vi "View.vi"(8 "error in (no error)":errorcluster, 11 "XY Stage Class in":refnum<class "XY Stage Class.lvclass">) -> (0 "error out":errorcluster, 3 "XY Stage Class out":refnum<class "XY Stage Class.lvclass">)   [LabVIEW 2022 SP3, in "XY Stage Class.lvclass"]
uses:
  XY Stage Class.lvclass
  C:/XY Stage/iView/base view/base view.lvclass
  Interfaces/2-Axis Stage API/2-Axis Stage Async API.lvclass
  XY Controller/XY Stage Controller/XY Stage Controller.lvclass
  C:/XY Stage/XY Stage/Interfaces/2-Axis Stage API/2-Axis Stage Async API.lvclass
  iView/base view/Accessors/Read Event Registration Refnum.vi
  iView/base view/Accessors/Read View Refnum.vi
  iView/base view/base view.lvclass
panel:
  in  "2-Axis Stage":refnum<class "2-Axis Stage Async API.lvclass">
  out "XY Position Graph":cluster{"X":dbl, "Y":dbl}[](graph)
  in  "Abort Motion":bool
  in  "Home Stage":bool
  in  "Move Stage":bool
  in  "Y-Destination":dbl min=-100.0 max=100.0
  in  "X-Destination":dbl min=-100.0 max=100.0
  in  "Clear Error":bool
  in  "Set X-Speed":u16
  in  "Set Y-Speed":u16
  in  "Set X-Acceleration":u16
  in  "Set Y-Acceleration":u16
  out "X-Speed":dbl
  out "Y-Speed":dbl
  out "X-Current Speed":dbl
  out "Y-Current Speed":dbl
  out "X-Acceleration":dbl
  out "Y-Acceleration":dbl
  out "Y-Homed":bool
  out "X-Homed":bool
  out "X-Moving":bool
  out "Y-Moving":bool
  out "Y-Position":dbl
  out "X-Position":dbl
  out "Stage Error":errorcluster
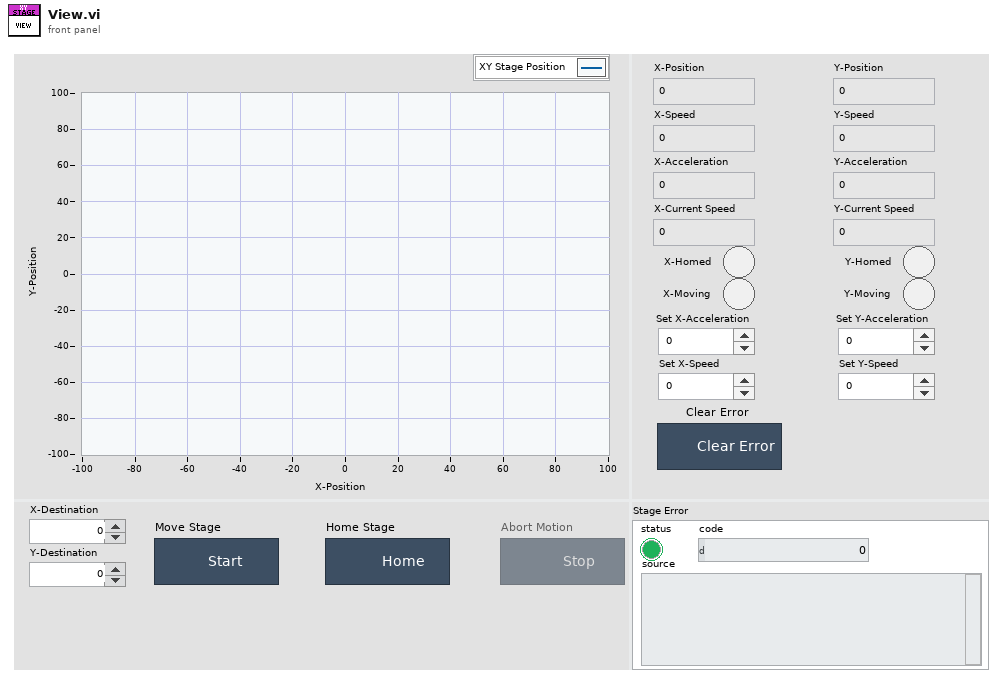
[diagram p1: front panel]
types:
  T1 = typedef "base view.lvclass/Events.ctl" = cluster{"Open":refnum<user-event>, "Close":refnum<user-event>, "Hide":refnum<user-event>}
  T2 = enum32{"Invalid", "Standard", "Closed", "Hidden", "Minimized", "Maximized"}
  T3 = enum32{"invalid app kind", "Development System", "Run Time System", "Student Edition", "Embedded LabVIEW", "Evaluation", "Custom"}
  T4 = enum8{"Enabled", "Disabled", "Disabled and Grayed Out"}
  T5 = cluster{"Current Position X":dbl, "Current Position Y":dbl}[]
  T6 = cluster{"Core":cluster{"Current VI Reference":refnum<vi>, "Close Panel on Exit?":bool}, "2-Axis Stage":refnum<class "2-Axis Stage Async API.lvclass">}
  T7 = cluster{"Current VI Reference":refnum<vi>, "Close Panel on Exit?":bool}
  T8 = cluster{"Event Registration Refnum":refnum<event-registration>, "Event Registration Refnum":refnum<event-registration>}
  T9 = cluster{"Event Registration Refnum":refnum<event-registration>, "Event Registration Refnum":refnum<event-registration>, "Event Registration Refnum":refnum<event-registration>}
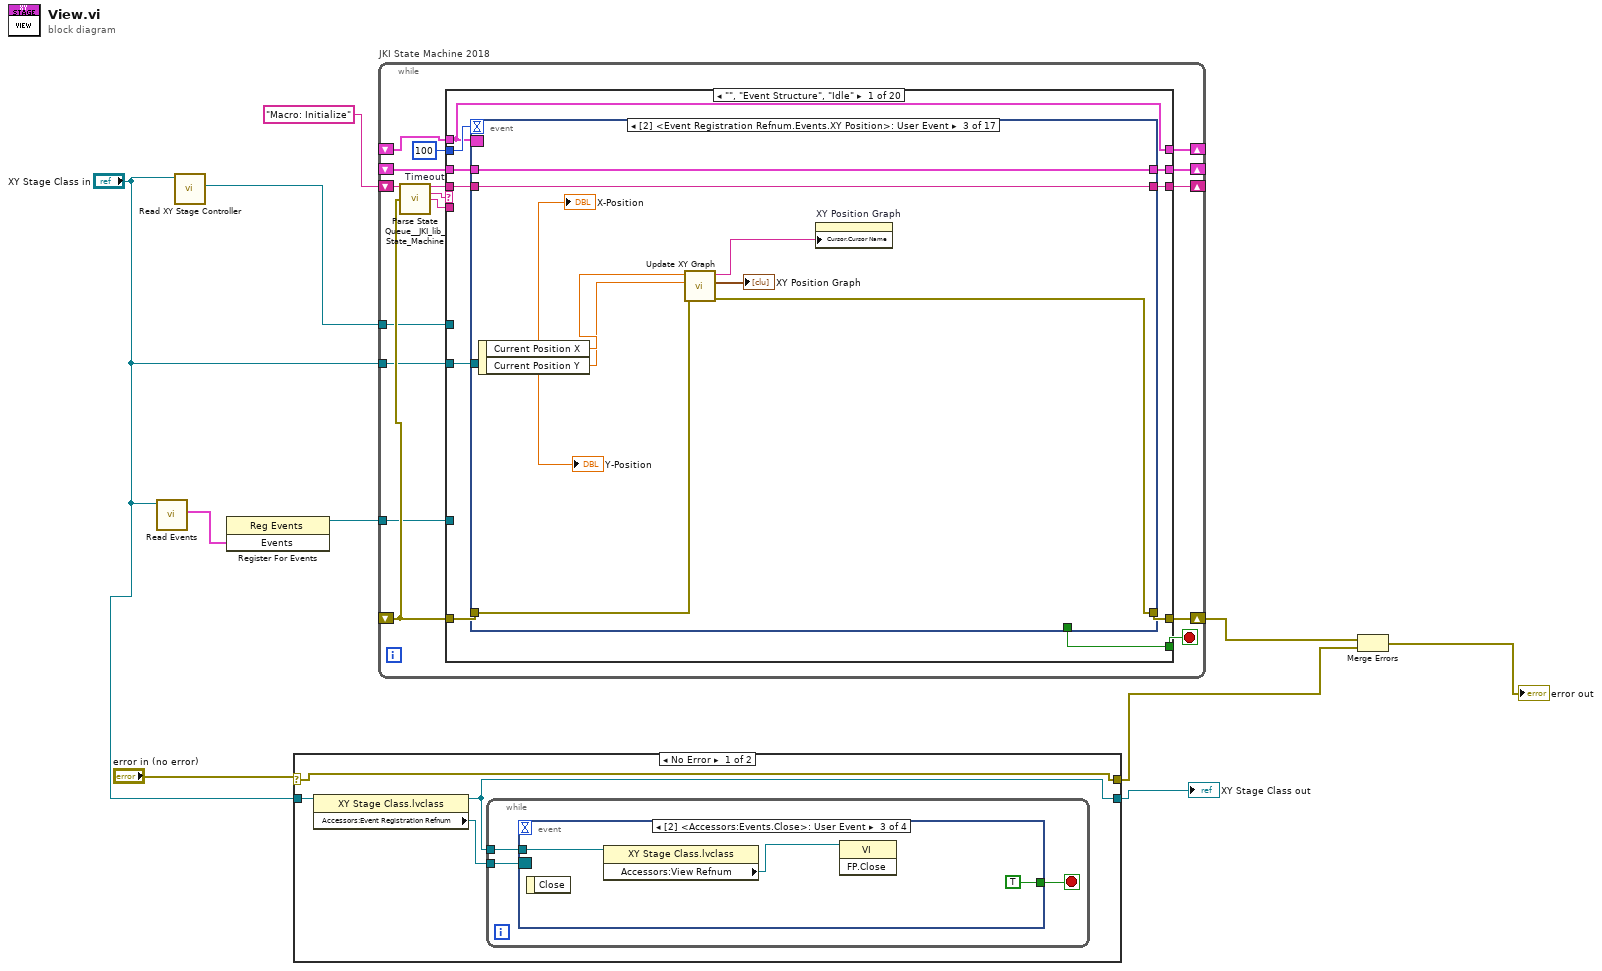
[diagram p0: block diagram]
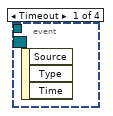
[diagram p2: hidden frame]
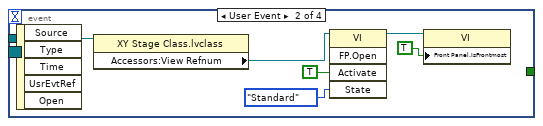
[diagram p3: hidden frame]
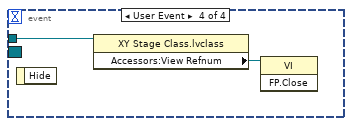
[diagram p4: hidden frame]
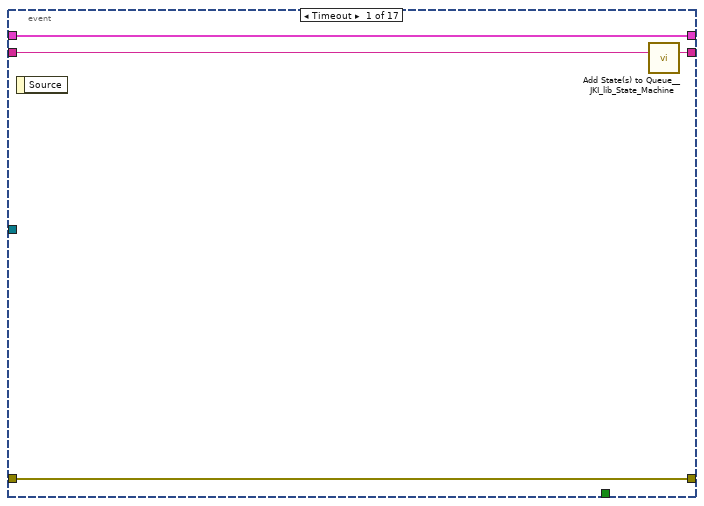
[diagram p6: hidden frame]
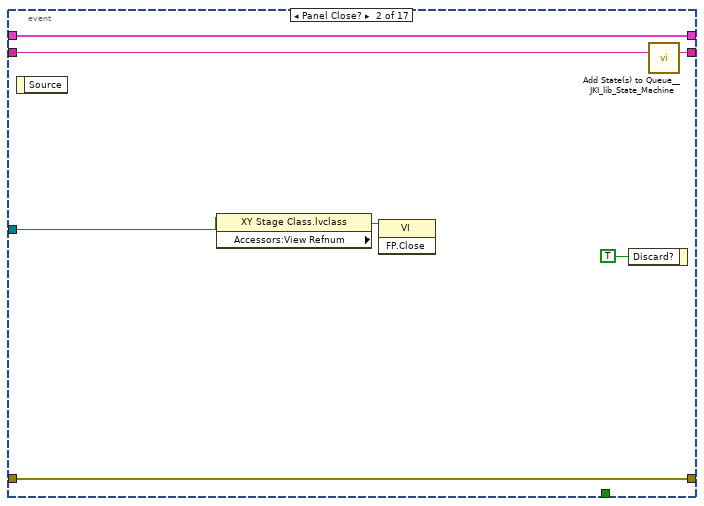
[diagram p7: hidden frame]
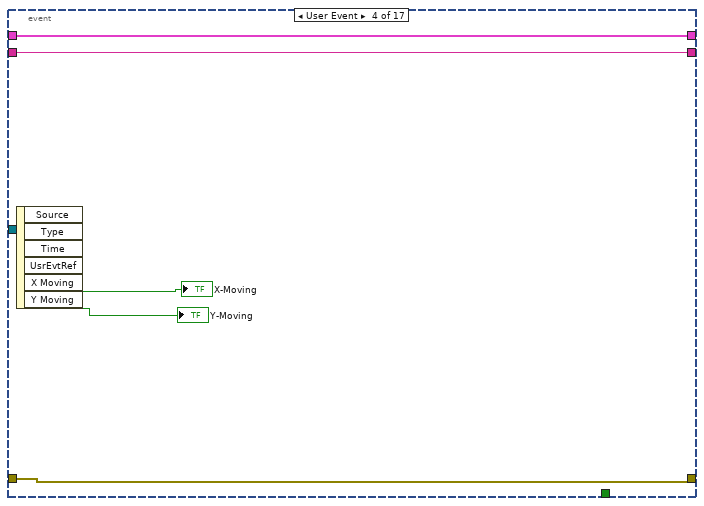
[diagram p8: hidden frame]
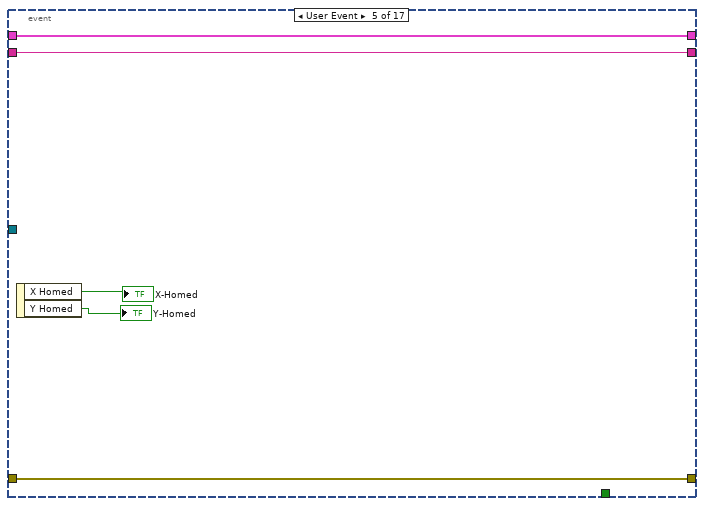
[diagram p9: hidden frame]
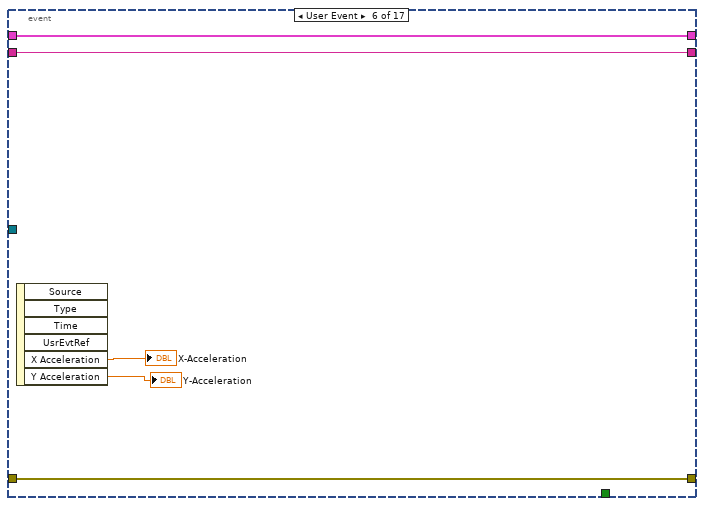
[diagram p10: hidden frame]
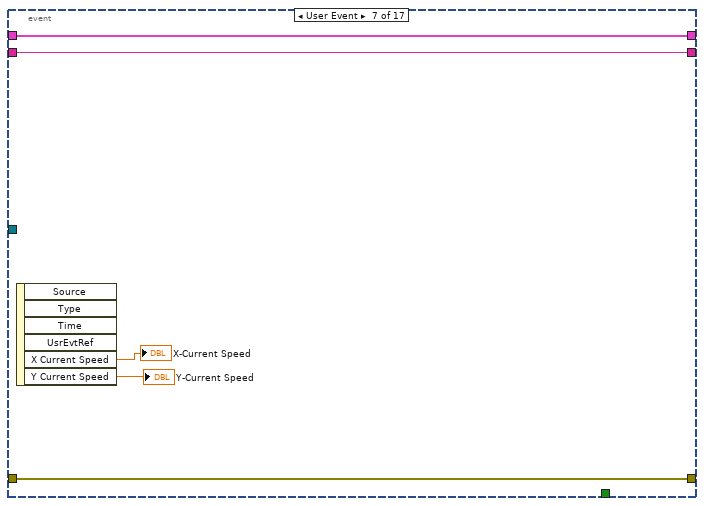
[diagram p11: hidden frame]
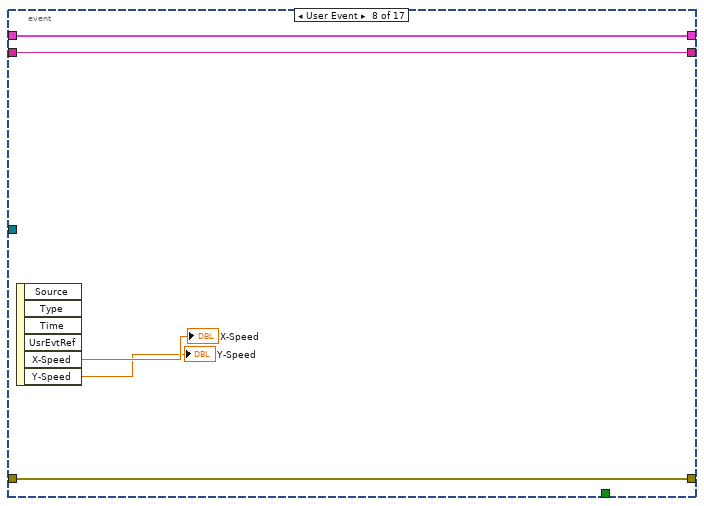
[diagram p12: hidden frame]
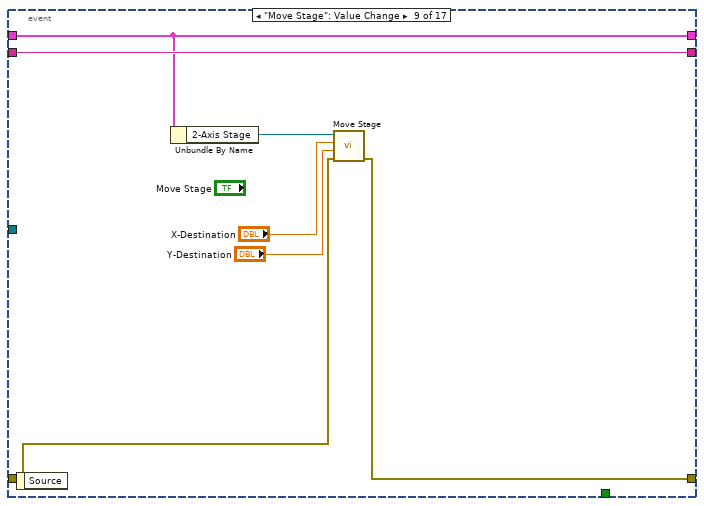
[diagram p13: hidden frame]
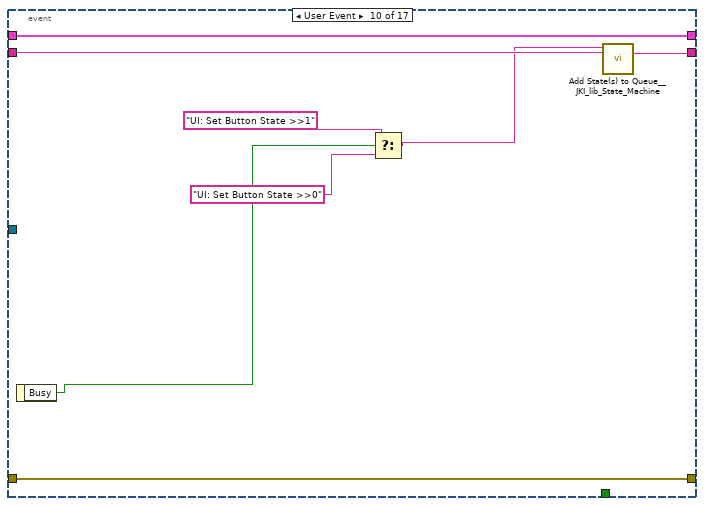
[diagram p14: hidden frame]
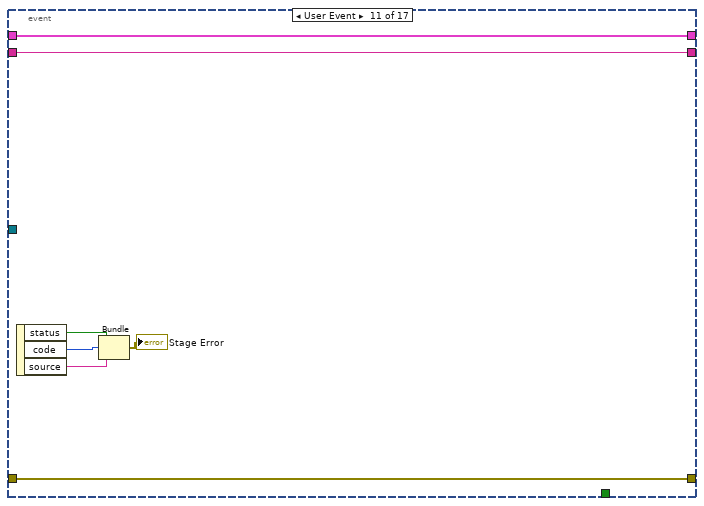
[diagram p15: hidden frame]
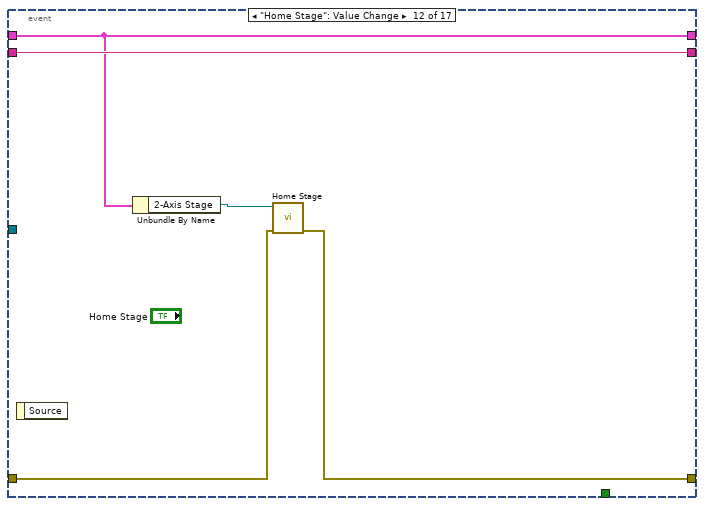
[diagram p16: hidden frame]
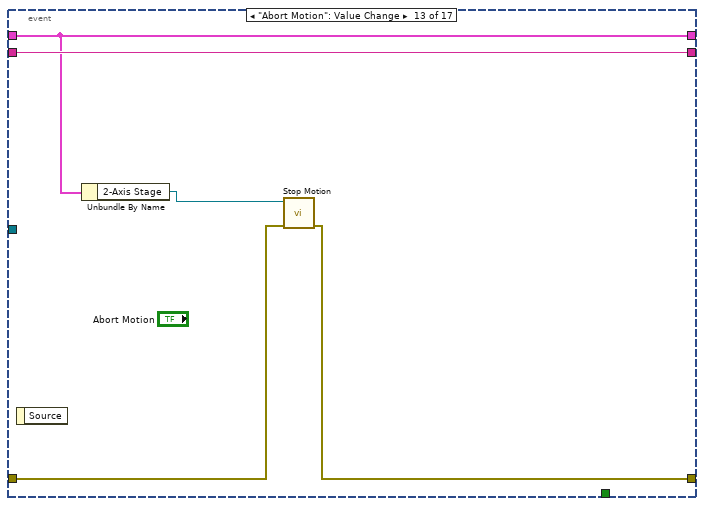
[diagram p17: hidden frame]
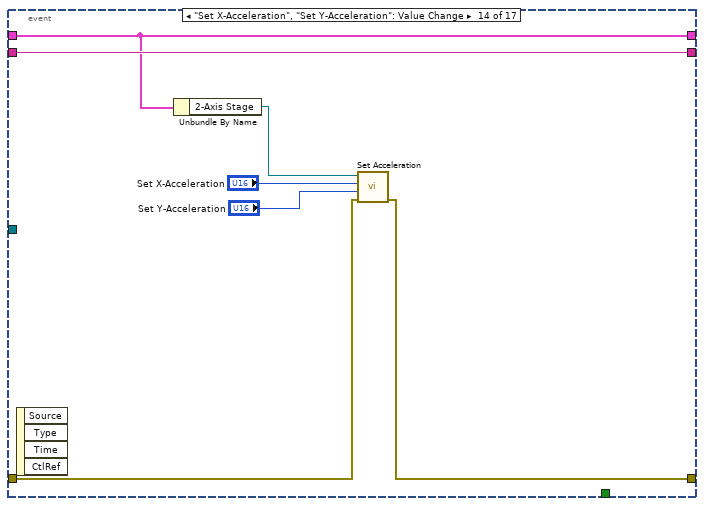
[diagram p18: hidden frame]
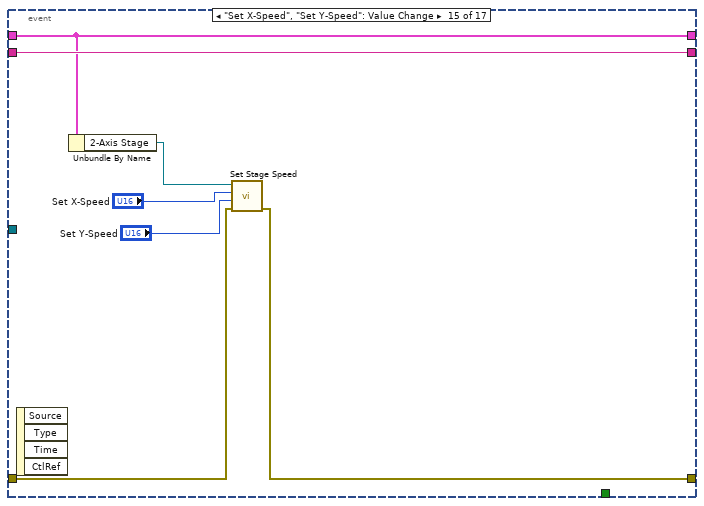
[diagram p19: hidden frame]
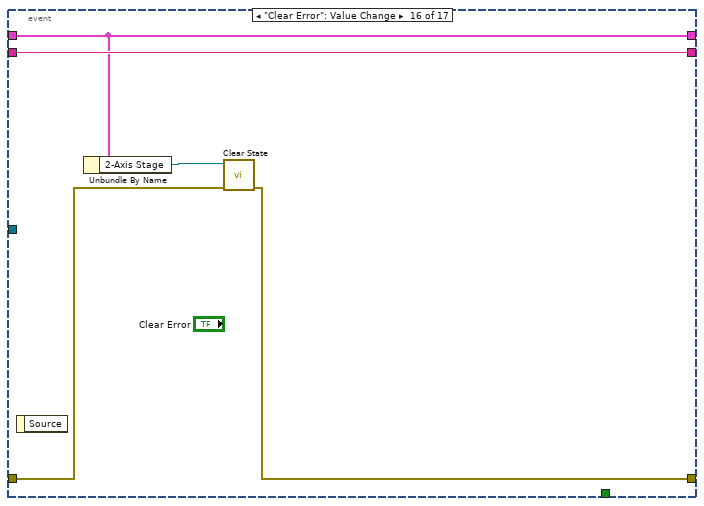
[diagram p20: hidden frame]
diagram:
  n1 = call "Read Events.vi"("In"="XY Stage Class in") -> ("Events"=w7:T1)  [unwired: 8 in, 2 out]
  n2 = call "Read XY Stage Controller.vi"("In"="XY Stage Class in") -> ("XY Stage Controller"=w8:refnum<class "XY Stage Controller.lvclass">)  [unwired: 8 in, 2 out]
  n3 = register-events(w7) -> (reference out=w6:refnum<event-registration>)  [unwired: 2 in, 1 out]
  n4 = case shown="No Error" "error in (no error)" {
    selector: "error in (no error)" -> [w14 w30]
    tunnel: [w14 w30] -> w3
    tunnel: [w11 w29] -> w10
    tunnel: "XY Stage Class in" -> [w13 w29]
    frame No Error {
      n5 = property class="XY Stage Class.lvclass"(reference=w13) -> (reference out=w11:refnum<class "XY Stage Class.lvclass">, "Accessors:Event Registration Refnum"=w12:refnum<event-registration>)  [unwired: 1 in, 1 out]
      n6 = while {
        tunnel: w12 -> [w17]
        tunnel: w11 -> [w15]
        stop <- w16 stop-if-true
        n7 = event shown="[2] <Accessors:Events.Close>: User Event" {
          selector: w17 -> [_ _ _ _]
          dyn-events: _ -> [_ _ _ _]
          timeout: _ -> [_ _ _ _]
          tunnel: [_ _ TRUE _] -> w16
          tunnel: w15 -> [_ w23 w24 w28]
          event Timeout {
            n8 = event-data() -> ()  [unwired: 1 in, 3 out]
          }
          event User Event {
            n9 = event-data() -> ()  [unwired: 1 in, 5 out]
            n10 = property class="XY Stage Class.lvclass"(reference=w23) -> ("Accessors:View Refnum"=w22:refnum<vi>)  [unwired: 1 in, 2 out]
            n11 = invoke class="VI" method="FP.Open"(reference=w22, "Activate"=TRUE ("Activate?"), "State"=T2."Standard") -> (reference out=w19:refnum<vi>)  [unwired: 2 in, 4 out]
            n12 = property class="VI"(reference=w19, "Front Panel.IsFrontmost"=TRUE ("Front Panel Window:Is Frontmost")) -> ()  [unwired: 1 in, 2 out]
          }
          event User Event {
            n13 = event-data() -> ()  [unwired: 1 in, 1 out]
            n14 = property class="XY Stage Class.lvclass"(reference=w24) -> ("Accessors:View Refnum"=w25:refnum<vi>)  [unwired: 1 in, 2 out]
            n15 = invoke class="VI" method="FP.Close"(reference=w25) -> ()  [unwired: 2 in, 3 out]
          }
          event User Event {
            n16 = event-data() -> ()  [unwired: 1 in, 1 out]
            n17 = property class="XY Stage Class.lvclass"(reference=w28) -> ("Accessors:View Refnum"=w27:refnum<vi>)  [unwired: 1 in, 2 out]
            n18 = invoke class="VI" method="FP.Close"(reference=w27) -> ()  [unwired: 2 in, 3 out]
          }
        }
      }
    }
    frame Error {
    }
  }
  "XY Stage Class out" <- w10
  n19 = while "JKI State Machine 2018" {
    shift-right: [w39] -> _
    shift-left: _ -> [w38]
    shift-right: [w42] -> w4
    shift-left: _ -> [w36]
    shift-right: [w41] -> _
    shift-left: "Macro: Initialize" -> [w43]
    shift-right: [w35] -> _
    shift-left: _ -> [w34]
    tunnel: w8 -> [w33]
    tunnel: w6 -> [w32]
    tunnel: "XY Stage Class in" -> [w31]
    stop <- w40 stop-if-true
    w37 = 100  # Timeout
    n20 = call <vilib>:"Parse State Queue__JKI_lib_State_Machine.vi"("State Queue"=w43, "Error In (no error)"=w36) -> ("Remaining States"=w45:string, "Current State"=w46:string, "Arguments"=w44:string)  [unwired: 11 in]
    n21 = case shown="\"\", \"Event Structure\", \"Idle\"" w46 {
      selector: w46 -> [_ _ w162 _ _ _ _ _ _ _ _ _ _ _ _ _ _ _ _ _]
      tunnel: w45 -> [w56 w160 w166 w186 w193 w199 w204 w213 w220 w225 w248 w259 w291 w313 w325 w395 w401 w412 w417 w427]
      tunnel: w44 -> [_ _ _ _ _ _ _ _ _ _ _ _ w280 w308 w319 _ _ _ _ _]
      tunnel: w38 -> [w54 w157 w164 w179 w190 w197 w201 _ w215 w222 w245 w263 w282 w311 w321 w392 w398 w409 w414 w426]
      tunnel: [w53 w158 w168 w183 errorcluster {"status"=FALSE, "code"=0, "source"=""} ("error out") w196 w202 w210 w216 w223 w230 w254 w277 w309 w322 w393 w399 w410 w415 w423] -> w42
      tunnel: w36 -> [w52 w158 w167 w183 w187 w196 w202 w210 w217 w223 w237 w261 w276 w310 w323 w393 w399 w410 w415 w424]
      tunnel: [w55 w159 w165 w185 w192 w198 w203 w212 w219 w224 w247 w260 w291 w312 w324 w394 w400 w411 w416 w427] -> w41
      tunnel: [w48 _ _ _ _ TRUE _ _ _ _ _ _ _ _ _ _ _ _ _ _] -> w40
      tunnel: [w51 w157 w164 w184 w190 w197 w201 w206 w215 w222 w245 w263 w282 w311 w321 w392 w398 w409 w414 w426] -> w39
      tunnel: w37 -> [w50 _ _ _ _ _ _ _ _ _ _ _ _ _ _ _ _ _ _ _]
      tunnel: [w49 w156 w161 w173 w188 w194 w200 w207 w214 w221 w246 w274 w283 w307 w318 w391 w397 w402 w413 w421] -> w35
      tunnel: w34 -> [w49 w156 w161 w173 w188 w194 w200 w207 w214 w221 w246 w274 w283 w307 w318 w391 w397 w402 w413 _]
      tunnel: w33 -> [_ _ _ _ _ _ _ w205 _ _ _ _ _ _ _ _ _ _ _ _]
      tunnel: w32 -> [_ _ _ _ _ _ _ _ _ _ _ _ _ _ _ _ _ _ _ w422]
      tunnel: w31 -> [w47 _ _ _ _ _ _ _ _ _ _ _ _ _ _ _ _ _ _ _]
      frame "", "Event Structure", "Idle" {
        n22 = event shown="[2] <Event Registration Refnum.Events.XY Position>: User Event" {
          selector: w49 -> [_ _ _ _ _ _ _ _ _ _ _ _ _ _ _ _ _]
          dyn-events: _ -> [_ _ _ _ _ _ _ _ _ _ _ _ _ _ _ _ _]
          timeout: w50 -> [_ _ _ _ _ _ _ _ _ _ _ _ _ _ _ _ _]
          tunnel: w56 -> [w60 w67 w74 w80 w85 w90 w95 w100 w107 w112 w122 w127 w132 w139 w146 w151 w155]
          tunnel: [w59 w66 w74 w80 w85 w90 w95 w100 w107 w113 w122 w127 w132 w139 w146 w151 w155] -> w55
          tunnel: w54 -> [w57 w64 w75 w79 w84 w89 w94 w99 w106 w115 w121 w126 w131 w138 w145 w150 w154]
          tunnel: [w58 w65 w68 w76 w81 w86 w91 w96 w101 w114 w116 w123 w129 w133 w142 w147 w152] -> w53
          tunnel: w52 -> [w58 w65 w69 w76 w81 w86 w91 w96 w102 w114 w116 w124 w128 w134 w143 w148 w152]
          tunnel: [w57 w64 w75 w79 w84 w89 w94 w99 w106 w115 w121 w126 w131 w138 w145 w150 w154] -> w51
          tunnel: [_ _ _ _ _ _ _ _ _ _ _ _ _ _ _ _ TRUE] -> w48
          tunnel: w47 -> [_ w61 _ _ _ _ _ _ _ _ _ _ _ _ _ _ _]
          event Timeout {
            n23 = event-data() -> ()  [unwired: 1 in, 1 out]
            n24 = call <vilib>:"Add State(s) to Queue__JKI_lib_State_Machine.vi"("State(s) in (\"\")"=w60) -> ("States Out"=w59:string)  [unwired: 14 in]
          }
          event Panel Close? {
            n25 = event-data() -> ()  [unwired: 1 in, 1 out]
            n26 = property class="XY Stage Class.lvclass"(reference=w61) -> ("Accessors:View Refnum"=w62:refnum<vi>)  [unwired: 1 in, 2 out]
            n27 = invoke class="VI" method="FP.Close"(reference=w62) -> ()  [unwired: 2 in, 3 out]
            n28 = event-data("Discard?"=TRUE) -> ()  [unwired: 1 in, 1 out]
            n29 = call <vilib>:"Add State(s) to Queue__JKI_lib_State_Machine.vi"("State(s) in (\"\")"=w67) -> ("States Out"=w66:string)  [unwired: 14 in]
          }
          event User Event {
            n30 = event-data() -> ("Current Position X"=w72:dbl, "Current Position Y"=w71:dbl)  [unwired: 1 in]
            "Y-Position" <- w71
            "X-Position" <- w72
            n31 = call "Update XY Graph.vi"("error in (no error)"=w69, "Current Position Y"=w71, "Current Position X"=w72) -> ("error out"=w68:errorcluster, "Array"=→"XY Position Graph":T5, "String"=w70:string)  [unwired: 6 in]
            n32 = property on="XY Position Graph" class="XYGraph (strict)"("Cursor.Cursor Name"=w70) -> ()  [unwired: 2 in, 2 out]
          }
          event User Event {
            n33 = event-data() -> ("X Moving"=→"X-Moving":bool, "Y Moving"=→"Y-Moving":bool)  [unwired: 1 in, 4 out]
          }
          event User Event {
            n34 = event-data() -> ("X Homed"=→"X-Homed":bool, "Y Homed"=→"Y-Homed":bool)  [unwired: 1 in]
          }
          event User Event {
            n35 = event-data() -> ("X Acceleration"=→"X-Acceleration":dbl, "Y Acceleration"=→"Y-Acceleration":dbl)  [unwired: 1 in, 4 out]
          }
          event User Event {
            n36 = event-data() -> ("X Current Speed"=→"X-Current Speed":dbl, "Y Current Speed"=→"Y-Current Speed":dbl)  [unwired: 1 in, 4 out]
          }
          event User Event {
            n37 = event-data() -> ("X-Speed"=→"X-Speed":dbl, "Y-Speed"=→"Y-Speed":dbl)  [unwired: 1 in, 4 out]
          }
          event "Move Stage": Value Change {
            n38 = event-data() -> ()  [unwired: 1 in, 1 out]
            n39 = Unbundle By Name(w106) -> ("2-Axis Stage"=w105:refnum<class "2-Axis Stage Async API.lvclass">)
            n40 = call-dynamic "Move Stage.vi"("error in (no error)"=w102, "Y Axis"="Y-Destination", "X Axis"="X-Destination", "2-Axis Stage in"=w105) -> ("error out"=w101:errorcluster)  [unwired: 6 in, 1 out]
          }
          event User Event {
            n41 = event-data() -> ("Busy"=w111:bool)  [unwired: 1 in]
            n42 = Select(t="UI: Set Button State >>1", s=w111, f="UI: Set Button State >>0") -> (s? t:f=w108:string)
            n43 = call <vilib>:"Add State(s) to Queue__JKI_lib_State_Machine.vi"("State(s) in Front (\"\")"=w108, "State(s) in (\"\")"=w112) -> ("States Out"=w113:string)  [unwired: 13 in]
          }
          event User Event {
            n44 = event-data() -> ("status"=w120:bool, "code"=w119:i32, "source"=w118:string)  [unwired: 1 in]
            n45 = Bundle("status"=w120, "code"=w119, "source"=w118) -> (→"Stage Error":errorcluster)  [unwired: 1 in]
          }
          event "Home Stage": Value Change {
            n46 = event-data() -> ()  [unwired: 1 in, 1 out]
            n47 = Unbundle By Name(w126) -> ("2-Axis Stage"=w125:refnum<class "2-Axis Stage Async API.lvclass">)
            n48 = call-dynamic "Home Stage.vi"("error in (no error)"=w124, "2-Axis Async Home in"=w125) -> ("error out"=w123:errorcluster)  [unwired: 8 in, 1 out]
          }
          event "Abort Motion": Value Change {
            n49 = event-data() -> ()  [unwired: 1 in, 1 out]
            n50 = Unbundle By Name(w131) -> ("2-Axis Stage"=w130:refnum<class "2-Axis Stage Async API.lvclass">)
            n51 = call-dynamic "Stop Motion.vi"("error in (no error)"=w128, "2-Axis Stage in"=w130) -> ("error out"=w129:errorcluster)  [unwired: 8 in, 1 out]
          }
          event "Set X-Acceleration", "Set Y-Acceleration": Value Change {
            n52 = event-data() -> ()  [unwired: 1 in, 4 out]
            n53 = Unbundle By Name(w138) -> ("2-Axis Stage"=w137:refnum<class "2-Axis Stage Async API.lvclass">)
            n54 = call-dynamic "Set Acceleration.vi"("error in (no error)"=w134, "Y Axis"="Set Y-Acceleration", "X Axis"="Set X-Acceleration", "2-Axis Stage in"=w137) -> ("error out"=w133:errorcluster)  [unwired: 6 in, 1 out]
          }
          event "Set X-Speed", "Set Y-Speed": Value Change {
            n55 = event-data() -> ()  [unwired: 1 in, 4 out]
            n56 = Unbundle By Name(w145) -> ("2-Axis Stage"=w144:refnum<class "2-Axis Stage Async API.lvclass">)
            n57 = call-dynamic "Set Stage Speed.vi"("error in (no error)"=w143, "Y Axis"="Set Y-Speed", "X Axis"="Set X-Speed", "2-Axis Stage in"=w144) -> ("error out"=w142:errorcluster)  [unwired: 6 in, 1 out]
          }
          event "Clear Error": Value Change {
            n58 = event-data() -> ()  [unwired: 1 in, 1 out]
            n59 = Unbundle By Name(w150) -> ("2-Axis Stage"=w149:refnum<class "2-Axis Stage Async API.lvclass">)
            n60 = call-dynamic "Clear State.vi"("error in (no error)"=w148, "2-Axis Stage Status in"=w149) -> ("error out"=w147:errorcluster)  [unwired: 8 in, 1 out]
          }
          event User Event {
            n61 = event-data() -> ()  [unwired: 1 in, 1 out]
          }
        }
      }
      frame "---------- Core ----------" {
        # "Do not put any code in this frame.\n(it is a separator no-op)"
        n62 = call <vilib>:"Add State(s) to Queue__JKI_lib_State_Machine.vi"("State(s) in (\"\")"=w160) -> ("States Out"=w159:string)  [unwired: 14 in]
      }
      frame Default {
        w171 = 42 items=["No error", "Argument error", "Memory is full", "Out of zone", "End of file", "File already open", "Generic file I/O error", "File not found", "File permission error", "Disk is full", "Duplicate path", "Too many files open", "System feature not enabled", "Resource file not found", "Cannot add resource", "Resource not found", "Image not found", "Image memory error", "Pen does not exist", "Config type invalid", "Config token not found", "Config parse error", "Config memory error", "Bad external code format", "Bad external code offset", "External code not present", "Null window", "Destroy window error", "Null menu", "Print aborted", "Bad print record", "Print driver error", "Windows error during printing", "Memory error during printing", "Print dialog error", "Generic print error", "Invalid device refnum", "Device not found", "Device parameter error", "Device unit error", "Cannot open device", "Device call aborted", "Generic error", "Cancelled by user", "Object ID too low", "Object ID too high", "Object not in heap", "Unknown heap", "Unknown object (invalid DefProc)", "Unknown object (DefProc not in table)", "Message out of range", "Invalid (null) method", "Unknown message", "Manager call not supported", "Bad address", "Network operation in progress", "Network operation timed out", "Connection is busy", "Network attribute not supported", "Network error", "Address in use", "System out of memory", "Connection aborted", "Connection refused", "Not connected", "Already connected", "Connection closed", "Initialization error (interapplication manager)", "Bad occurrence", "Wait on unbound occurrence handler", "Occurrence queue overflow", "Datalog type conflict", "Unused", "Unrecognized type (interapplication manager)", "Memory corrupt", "Failed to make temporary DLL", "Old CIN version", "Drag socket not found", "Failed to load drop-object", "Failed to register OLE object", "Failed to release OLE object", "Format specifier type mismatch", "Unknown format specifier", "Too few format specifiers", "Too many format specifiers", "Scan failed", "Newer CIN version", "Error converting to variant", "Runtime menu error", "Password tampered", "Variant attribute not found", "Incompatible variant data type", "Event data is not available", "Event Store is not present", "Occurrence is not found", "Event Queue is not created", "Event info is not available", "Refnum passed is NULL", "Error retrieving Class GUID", "Error retrieving CoClass GUID", "Error retrieving TypeLib GUID.", "Bad built application magic bytes.", "Specific driver is different from the specific driver associated with the Logical Name.", "There is no session opened to the class driver.", "Max Error", "MAX - Error with config objects", "MAX - Error loading configuration", "MAX - Group not supported"]
        # "Current State"
        # "Do not delete, rename, or modify this frame.\n(this is used to capture unhandled states and typos)"
        # "Handle mistyped state name (developer tool)"
        n63 = Format Into String(format string="Software Exception: Unhandled State \"%s\"." ("message"), error in=w167, w162) -> (resulting string=w170:string, error out=w169:errorcluster)  [unwired: 1 in]
        n64 = call <vilib>:"Error Cluster From Error Code.vi"("show call chain? (False)"=TRUE, "error in (no error)"=w169, "error message (\"\")"=w170, "error code (0)"=w171) -> ("error out"=w168:errorcluster)  [unwired: 5 in]
        n65 = call <vilib>:"Add State(s) to Queue__JKI_lib_State_Machine.vi"("State(s) in (\"\")"=w166) -> ("States Out"=w165:string)  [unwired: 14 in]
      }
      frame "Initialize Core Data" {
        # "Do not delete, rename, or modify this frame.\n(this is used to determine panel behavior on exit)"
        # "originally closed?"
        # "exe?"
        # "If panel starts closed or is an EXE, then close it when we exit"
        n66 = property class="VI"() -> ("FP.State"=w176:T2)  [unwired: 2 in, 2 out]
        n67 = property class="App"() -> ("App.Kind"=w182:T3)  [unwired: 2 in, 2 out]
        n68 = control-ref of="Current VI Reference"() -> (w177:refnum<vi>)
        n69 = Equal?(x=w176, y=T2."Closed" ("Front Panel Window:State")) -> (x = y?=w174:bool)
        n70 = Equal?(x=w182, y=T3."Run Time System" ("Application:Kind")) -> (x = y?=w180:bool)
        n71 = Or(x=w174, y=w180) -> (x .or. y?=w178:bool)
        n72 = Bundle By Name(cluster=w179, "Core.Current VI Reference"=w177, "Core.Close Panel on Exit?"=w178) -> (w184:T6)
        n73 = call <vilib>:"Add State(s) to Queue__JKI_lib_State_Machine.vi"("State(s) in (\"\")"=w186) -> ("States Out"=w185:string)  [unwired: 14 in]
      }
      frame "Error Handler" {
        # "Handle any errors here.\nYou can also output any states to clean-up after errors occur"
        # "Clear error"
        n74 = local write "Stage Error"(w187) -> ()
        n75 = call <vilib>:"Add State(s) to Queue__JKI_lib_State_Machine.vi"("State(s) in Front (\"\")"="/* Post Error States", "State(s) in (\"\")"=w193) -> ("States Out"=w192:string)  [unwired: 13 in]
      }
      frame "Exit" {
        # "Do not put any code in this frame.\n(No errors that occur here will be handled.)"
        n76 = call <vilib>:"Add State(s) to Queue__JKI_lib_State_Machine.vi"("State(s) in (\"\")"=w199) -> ("States Out"=w198:string)  [unwired: 14 in]
      }
      frame "---------- Data ----------" {
        # "Do not put any code in this frame.\n(It is a separator no-op. You can make a copy of this frame to create a new Data frame)"
        n77 = call <vilib>:"Add State(s) to Queue__JKI_lib_State_Machine.vi"("State(s) in (\"\")"=w204) -> ("States Out"=w203:string)  [unwired: 14 in]
      }
      frame "Data: Initialize" {
        w209 = T7 {"Current VI Reference"=refnum, "Close Panel on Exit?"=FALSE}  # Core
        # "Data names and types of shift register data are defined by this bundle."
        # "Initialize the shift-register data, here.\n(data names are defined by what you wire into the bundle function)"
        n78 = Bundle("Core"=w209, "2-Axis Stage"="2-Axis Stage") -> (w211:T6)  [unwired: 1 in]
        n79 = Bundle By Name(cluster=w211, "2-Axis Stage"=w205) -> (w206:T6)
        n80 = call <vilib>:"Add State(s) to Queue__JKI_lib_State_Machine.vi"("State(s) in (\"\")"=w213) -> ("States Out"=w212:string)  [unwired: 14 in]
      }
      frame "Data: Cleanup" {
        # "Cleanup any data and references, here.\n(this is called automatically, by the Macro: Exit)"
        n81 = Unbundle By Name(w215) -> ("Core.Current VI Reference"=w218:refnum<vi>)
        n82 = Close Reference(reference=w218, error in (no error)=w217) -> (error out=w216:errorcluster)
        n83 = call <vilib>:"Add State(s) to Queue__JKI_lib_State_Machine.vi"("State(s) in (\"\")"=w220) -> ("States Out"=w219:string)  [unwired: 14 in]
      }
      frame "---------- UI ----------" {
        # "Do not put any code in this frame.\n(It is a separator no-op. You can make a copy of this frame to create a new UI frame)"
        n84 = call <vilib>:"Add State(s) to Queue__JKI_lib_State_Machine.vi"("State(s) in (\"\")"=w225) -> ("States Out"=w224:string)  [unwired: 14 in]
      }
      frame "UI: Initialize 1" {
        # "Initialize the User Interface, here.\n(this is called automatically, by the Macro: Init)"
        n85 = Unbundle By Name(w245) -> ("2-Axis Stage"=w242:refnum<class "2-Axis Stage Async API.lvclass">)
        n86 = call-dynamic "Read Current Position.vi"("error in (no error)"=w237, "2-Axis Stage Status in"=w242) -> ("error out"=w239:errorcluster, "Y Position"=w228:dbl, "X Position"=w229:dbl, "2-Axis Stage Status out"=w241:refnum<class "2-Axis Stage Async API.lvclass">)  [unwired: 6 in]
        n87 = call "Update XY Graph.vi"("Current Position Y"=w228, "Current Position X"=w229) -> ("Array"=w227:T5, "String"=w226:string)  [unwired: 7 in, 1 out]
        n88 = local write "X-Position"(w229) -> ()
        n89 = local write "Y-Position"(w228) -> ()
        n90 = local write "XY Position Graph"(w227) -> ()
        n91 = property on="XY Position Graph" class="XYGraph (strict)"("Cursor.Cursor Name"=w226) -> ()  [unwired: 2 in, 2 out]
        n92 = call-dynamic "Read Moving Flags.vi"("error in (no error)"=w239, "2-Axis Stage Status in"=w241) -> ("error out"=w238:errorcluster, "Y-Axis Moving"=w243:bool, "X-Axis Moving"=w244:bool, "2-Axis Stage Status out"=w240:refnum<class "2-Axis Stage Async API.lvclass">)  [unwired: 6 in]
        n93 = local write "Y-Moving"(w243) -> ()
        n94 = local write "X-Moving"(w244) -> ()
        n95 = call-dynamic "Read Stage Homed.vi"("error in (no error)"=w238, "2-Axis Stage Status in"=w240) -> ("error out"=w230:errorcluster, "Y-Axis Homed"=w235:bool, "X-Axis Homed"=w236:bool)  [unwired: 6 in, 1 out]
        n96 = local write "Y-Homed"(w235) -> ()
        n97 = And(x=w236, y=w235) -> (x .and. y?=w234:bool)
        n98 = Select(t=T4."Enabled" ("Disabled"), s=w234, f=T4."Disabled and Grayed Out" ("Disabled")) -> (s? t:f=w232:T4)
        n99 = local write "X-Homed"(w236) -> ()
        n100 = property on="Move Stage" class="Bool"("DisabledEnum"=w232) -> ()  [unwired: 2 in, 2 out]
        n101 = call <vilib>:"Add State(s) to Queue__JKI_lib_State_Machine.vi"("State(s) in (\"\")"=w248) -> ("States Out"=w247:string)  [unwired: 14 in]
      }
      frame "UI: Initialize 2" {
        # "#DEV_NOTES Need to read cache everytime VieW comes up. Cannot rely on just events since they only publish when there is change"
        n102 = Unbundle By Name(w263) -> ("2-Axis Stage"=w262:refnum<class "2-Axis Stage Async API.lvclass">, "Core.Current VI Reference"=w251:refnum<vi>)
        n103 = call-dynamic "Read Current Speed.vi"("error in (no error)"=w261, "2-Axis Stage Status in"=w262) -> ("error out"=w270:errorcluster, "Y Current Speed"=w273:dbl, "X Current Speed"=w272:dbl, "2-Axis Stage Status out"=w271:refnum<class "2-Axis Stage Async API.lvclass">)  [unwired: 6 in]
        n104 = local write "X-Current Speed"(w272) -> ()
        n105 = local write "Y-Current Speed"(w273) -> ()
        n106 = property class="VI"(reference=w251, "Front Panel.Title"="XY-Stage" ("Front Panel Window:Title"), "Front Panel.ShowMenuBar"=FALSE ("Front Panel Window:Show Menu Bar")) -> ()  [unwired: 1 in, 2 out]
        n107 = call-dynamic "Read Acceleration.vi"("error in (no error)"=w270, "2-Axis Stage Status in"=w271) -> ("error out"=w268:errorcluster, "Y Acceleration"=w264:dbl, "X Acceleration"=w265:dbl, "2-Axis Stage Status out"=w269:refnum<class "2-Axis Stage Async API.lvclass">)  [unwired: 6 in]
        n108 = local write "Set Y-Acceleration"(w264) -> ()
        n109 = local write "Y-Acceleration"(w264) -> ()
        n110 = local write "X-Acceleration"(w265) -> ()
        n111 = local write "Set X-Acceleration"(w265) -> ()
        n112 = call-dynamic "Read Speed.vi"("error in (no error)"=w268, "2-Axis Stage Status in"=w269) -> ("error out"=w255:errorcluster, "Y-Axis Speed"=w266:dbl, "X-Axis Speed"=w267:dbl, "2-Axis Stage Status out"=w256:refnum<class "2-Axis Stage Async API.lvclass">)  [unwired: 6 in]
        n113 = local write "Y-Speed"(w266) -> ()
        n114 = local write "Set X-Speed"(w267) -> ()
        n115 = local write "X-Speed"(w267) -> ()
        n116 = local write "Set Y-Speed"(w266) -> ()
        n117 = call-dynamic "Ready Busy Status.vi"("error in (no error)"=w255, "2-Axis Stage Status in"=w256) -> ("error out"=w254:errorcluster, "Busy"=w253:bool)  [unwired: 7 in, 1 out]
        n118 = Boolean To (0,1)(Boolean=w253) -> (0, 1=w252:i16)
        n119 = Format Into String(format string="UI: Set Button State >> %d", w252) -> (resulting string=w257:string)  [unwired: 2 in, 1 out]
        n120 = call <vilib>:"Add State(s) to Queue__JKI_lib_State_Machine.vi"("State(s) in Front (\"\")"=w257, "State(s) in (\"\")"=w259) -> ("States Out"=w260:string)  [unwired: 13 in]
      }
      frame "UI: Set Button State" {
        n121 = Scan From String(format string="%d", input string=w280, error in=w276) -> (error out=w275:errorcluster, output 1=w278:i32)  [unwired: 2 in, 2 out]
        n122 = Unbundle By Name(w282) -> ("2-Axis Stage"=w281:refnum<class "2-Axis Stage Async API.lvclass">)
        n123 = case shown="1" w278 {
          tunnel: [T4."Enabled" ("Disabled") w305] -> w290
          tunnel: [T4."Disabled and Grayed Out" ("Disabled") T4."Enabled" ("Disabled")] -> w289
          tunnel: [w296 w305] -> w288
          tunnel: [w295 w304] -> w277
          tunnel: [w294 w305] -> w287
          tunnel: [w294 w305] -> w286
          tunnel: [w294 w305] -> w285
          tunnel: [w294 w305] -> w284
          tunnel: w281 -> [w293 _]
          tunnel: w275 -> [w292 w304]
          frame 0, Default {
            w294 = T4."Enabled" ("Disabled")
            n124 = call-dynamic "Read Stage Homed.vi"("error in (no error)"=w292, "2-Axis Stage Status in"=w293) -> ("error out"=w295:errorcluster, "Y-Axis Homed"=w300:bool, "X-Axis Homed"=w301:bool)  [unwired: 6 in, 1 out]
            n125 = And(x=w301, y=w300) -> (x .and. y?=w299:bool)
            n126 = Select(t=T4."Enabled" ("Disabled"), s=w299, f=T4."Disabled and Grayed Out" ("Disabled")) -> (s? t:f=w296:T4)
          }
          frame 1 {
            w305 = T4."Disabled and Grayed Out" ("Disabled")
          }
        }
        n127 = property on="Abort Motion" class="Bool"("DisabledEnum"=w289) -> ()  [unwired: 2 in, 2 out]
        n128 = property on="Set Y-Speed" class="DigNum (strict)"("DisabledEnum"=w287) -> ()  [unwired: 2 in, 2 out]
        n129 = property on="Set X-Speed" class="DigNum (strict)"("DisabledEnum"=w286) -> ()  [unwired: 2 in, 2 out]
        n130 = property on="Set Y-Acceleration" class="DigNum (strict)"("DisabledEnum"=w285) -> ()  [unwired: 2 in, 2 out]
        n131 = property on="Set X-Acceleration" class="DigNum (strict)"("DisabledEnum"=w284) -> ()  [unwired: 2 in, 2 out]
        n132 = property on="Move Stage" class="Bool"("DisabledEnum"=w288) -> ()  [unwired: 2 in, 2 out]
        n133 = property on="Home Stage" class="Bool"("DisabledEnum"=w290) -> ()  [unwired: 2 in, 2 out]
      }
      frame "UI: Cursor Set" {
        # "Argument"
        # "Set and Unset Cursor Busy.\n(Usage: \"UI: Cursor Set >> Busy|Idle\")"
        n134 = case shown="\"Idle\", Default" w308 {
          tunnel: w310 -> [w315 w317]
          tunnel: [w314 w316] -> w309
          frame "Idle", Default {
            n135 = call <vilib>:"Unset Busy.vi"("error in (no error)"=w315) -> ("error out"=w314:errorcluster)  [unwired: 10 in]
          }
          frame "Busy" {
            n136 = call <vilib>:"Set Busy.vi"("error in (no error)"=w317) -> ("error out"=w316:errorcluster)  [unwired: 9 in, 1 out]
          }
        }
        n137 = call <vilib>:"Add State(s) to Queue__JKI_lib_State_Machine.vi"("State(s) in (\"\")"=w313) -> ("States Out"=w312:string)  [unwired: 14 in]
      }
      frame "UI: Front Panel State" {
        # "Argument"
        # "Set Front Panel Open or Closed\n(Usage: \"UI: Front Panel State >> Open|Close\")"
        n138 = Unbundle By Name(w321) -> ("Core.Current VI Reference"=w320:refnum<vi>)
        n139 = case shown="\"Minimize\", \"Minimized\"" w319 {
          tunnel: w323 -> [w331 w346 w357 w370 w383]
          tunnel: [w333 w347 w359 w372 w385] -> w322
          tunnel: w320 -> [w332 w344 w358 w371 w384]
          frame "Open", "Standard", Default {
            w326 = T2."Standard" ("State")
            n140 = property class="VI"(reference=w332, error in=w331) -> (reference out=w329:refnum<vi>, error out=w330:errorcluster, "FP.State"=w328:T2)
            n141 = Not Equal?(x=w328, y=w326) -> (x != y?=w327:bool)
            n142 = case shown="True" w327 {
              tunnel: [w337 w339] -> w333
              tunnel: w330 -> [w336 w339]
              tunnel: w329 -> [w335 _]
              tunnel: w326 -> [w334 _]
              frame True {
                n143 = invoke class="VI" method="FP.Open"(reference=w335, error in=w336, "Activate"=TRUE, "State"=w334) -> (error out=w337:errorcluster)  [unwired: 1 in, 4 out]
              }
              frame False {
              }
            }
          }
          frame "Close", "Closed" {
            n144 = property class="VI"(reference=w344, error in=w346) -> (reference out=w343:refnum<vi>, error out=w345:errorcluster, "FP.State"=w341:T2)
            n145 = Not Equal?(x=w341, y=T2."Closed" ("Front Panel Window:State")) -> (x != y?=w340:bool)
            n146 = case shown="True" w340 {
              tunnel: [w348 w351] -> w347
              tunnel: w345 -> [w348 w350]
              tunnel: w343 -> [_ w349]
              frame False {
              }
              frame True {
                n147 = invoke class="VI" method="FP.Close"(reference=w349, error in=w350) -> (error out=w351:errorcluster)  [unwired: 1 in, 2 out]
              }
            }
          }
          frame "Hidden", "Hide" {
            w352 = T2."Hidden" ("State")
            n148 = property class="VI"(reference=w358, error in=w357) -> (reference out=w355:refnum<vi>, error out=w356:errorcluster, "FP.State"=w354:T2)
            n149 = Not Equal?(x=w354, y=w352) -> (x != y?=w353:bool)
            n150 = case shown="True" w353 {
              tunnel: [w363 w364] -> w359
              tunnel: w356 -> [w362 w364]
              tunnel: w355 -> [w361 _]
              tunnel: w352 -> [w360 _]
              frame True {
                n151 = invoke class="VI" method="FP.Open"(reference=w361, error in=w362, "State"=w360) -> (error out=w363:errorcluster)  [unwired: 2 in, 4 out]
              }
              frame False {
              }
            }
          }
          frame "Minimize", "Minimized" {
            w365 = T2."Minimized" ("State")
            n152 = property class="VI"(reference=w371, error in=w370) -> (reference out=w368:refnum<vi>, error out=w369:errorcluster, "FP.State"=w367:T2)
            n153 = Not Equal?(x=w367, y=w365) -> (x != y?=w366:bool)
            n154 = case shown="True" w366 {
              tunnel: [w376 w377] -> w372
              tunnel: w369 -> [w375 w377]
              tunnel: w368 -> [w374 _]
              tunnel: w365 -> [w373 _]
              frame True {
                n155 = invoke class="VI" method="FP.Open"(reference=w374, error in=w375, "State"=w373) -> (error out=w376:errorcluster)  [unwired: 2 in, 4 out]
              }
              frame False {
              }
            }
          }
          frame "Maximize", "Maximized" {
            w378 = T2."Maximized" ("State")
            n156 = property class="VI"(reference=w384, error in=w383) -> (reference out=w381:refnum<vi>, error out=w382:errorcluster, "FP.State"=w380:T2)
            n157 = Not Equal?(x=w380, y=w378) -> (x != y?=w379:bool)
            n158 = case shown="True" w379 {
              tunnel: [w389 w390] -> w385
              tunnel: w382 -> [w388 w390]
              tunnel: w381 -> [w387 _]
              tunnel: w378 -> [w386 _]
              frame True {
                n159 = invoke class="VI" method="FP.Open"(reference=w387, error in=w388, "State"=w386) -> (error out=w389:errorcluster)  [unwired: 2 in, 4 out]
              }
              frame False {
              }
            }
          }
        }
        n160 = call <vilib>:"Add State(s) to Queue__JKI_lib_State_Machine.vi"("State(s) in (\"\")"=w325) -> ("States Out"=w324:string)  [unwired: 14 in]
      }
      frame "---------- Macro ----------" {
        # "Do not put any code in this frame.\n(It is a separator no-op. You can make a copy of this frame to create a new Macro frame)"
        n161 = call <vilib>:"Add State(s) to Queue__JKI_lib_State_Machine.vi"("State(s) in (\"\")"=w395) -> ("States Out"=w394:string)  [unwired: 14 in]
      }
      frame "Macro: Initialize" {
        w396 = "Data: Initialize\nInitialize Core Data\nEvents: Register for Events\nUI: Initialize 1\nUI: Initialize 2\nUI: Front Panel State >> Open"  # Data: Initialize Initialize Core Data Events: Register for Events UI: Initialize 1 UI: Initialize 2 UI: Front Panel State >> Open
        # "Initialization Macro\n(This is called once, when the VI starts)"
        n162 = call <vilib>:"Add State(s) to Queue__JKI_lib_State_Machine.vi"("State(s) in Front (\"\")"=w396, "State(s) in (\"\")"=w401) -> ("States Out"=w400:string)  [unwired: 13 in]
      }
      frame "Macro: Exit" {
        # "Exit Macro\n(This is called once, when the VI exits)"
        n163 = Unbundle By Name(w409) -> ("Core.Close Panel on Exit?"=w408:bool)
        n164 = Select(t="UI: Front Panel State >> Close", s=w408, f="") -> (s? t:f=w405:string)
        n165 = call <vilib>:"Add State(s) to Queue__JKI_lib_State_Machine.vi"("State(s) in (\"\")"=w405, "State(s) at Back (\"\")"="Data: Cleanup\nExit") -> ("States Out"=w403:string)  [unwired: 13 in]
        n166 = call <vilib>:"Add State(s) to Queue__JKI_lib_State_Machine.vi"("State(s) in Front (\"\")"=w403, "State(s) in (\"\")"=w412) -> ("States Out"=w411:string)  [unwired: 13 in]
      }
      frame "---------- Events ----------" {
        # "Template Separator\n(You can make a copy of, or modify, this frame)"
        n167 = call <vilib>:"Add State(s) to Queue__JKI_lib_State_Machine.vi"("State(s) in (\"\")"=w417) -> ("States Out"=w416:string)  [unwired: 14 in]
      }
      frame "Events: Register for Events" {
        n168 = Unbundle By Name(w426) -> ("2-Axis Stage"=w425:refnum<class "2-Axis Stage Async API.lvclass">)
        n169 = call-dynamic "Register for Events.vi"("error in (no error)"=w424, "Async Coms in"=w425) -> ("error out"=w423:errorcluster, "Event Refnums"=w420:T8)  [unwired: 7 in, 1 out]
        n170 = Unbundle By Name(w420) -> ("Event Registration Refnum"=w419:refnum<event-registration>, "Event Registration Refnum"=w418:refnum<event-registration>)
        n171 = Bundle("Event Registration Refnum"=w419, "Event Registration Refnum"=w418, "Event Registration Refnum"=w422) -> (w421:T9)  [unwired: 1 in]
      }
    }
  }
  n172 = Merge Errors(w4, w3) -> (→"error out":errorcluster)
